vi "Read Data Type.vi"(8 "error in (no error)":errorcluster, 11 "OnChange_Boolean in":refnum<class "OnChangeNotifier_Time.lvclass">) -> (0 "error out":errorcluster, 2 "Data Type":T1, 3 "OnChange_Boolean out":refnum<class "OnChangeNotifier_Time.lvclass">)   [LabVIEW 2021, in "OnChangeNotifier_Time.lvclass"]
uses:
  OnChangeNotifier_Time.lvclass
  Support/Class Type.ctl
  <vilib>/TSA/Abstract Data Classes/Abs_Types/Time/Abs_Time.lvclass
  OnChangeNotifier_Time.lvclass/OnChangeNotifier_Time.ctl
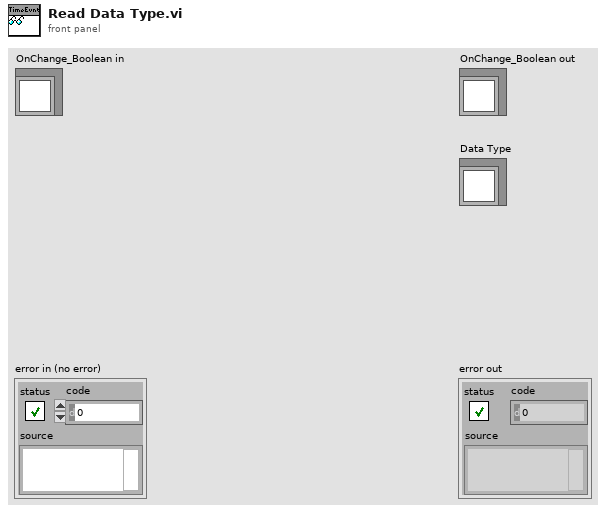
[diagram p1: front panel]
types:
  T1 = typedef "OnChangeNotifier_Time.lvclass/Class Type.ctl" = refnum<class "Abs_Time.lvclass">
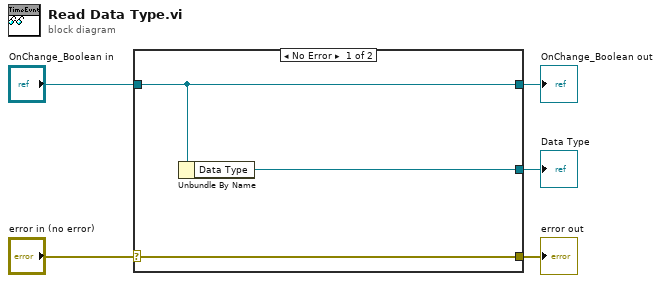
[diagram p0: block diagram]
diagram:
  n1 = case shown="No Error" "error in (no error)" {
    selector: "error in (no error)" -> [w8 w9]
    tunnel: [w8 w9] -> w4
    tunnel: [w7 w10] -> w2
    tunnel: "OnChange_Boolean in" -> [w7 w10]
    tunnel: [w6 _] -> w1
    frame No Error {
      n2 = Unbundle By Name(w7) -> ("Data Type"=w6:T1)
    }
    frame Error {
    }
  }
  "error out" <- w4
  "OnChange_Boolean out" <- w2
  "Data Type" <- w1
